vi "runLoopStop.vi"(8 "error in (no error)":errorcluster, 11 "Pixelfly in":refnum<class "Pixelfly.lvclass">) -> (0 "error out":errorcluster, 3 "Pixelfly out":refnum<class "Pixelfly.lvclass">)   [LabVIEW 2011, in "Hardware.lvlib" / "Channels.lvlib" / "Pixelfly.lvclass"]
uses:
  Pixelfly.lvclass
  Pixelfly.lvclass/Pixelfly.ctl
  Tools/Filing/FileSystem/FileSystem.lvclass
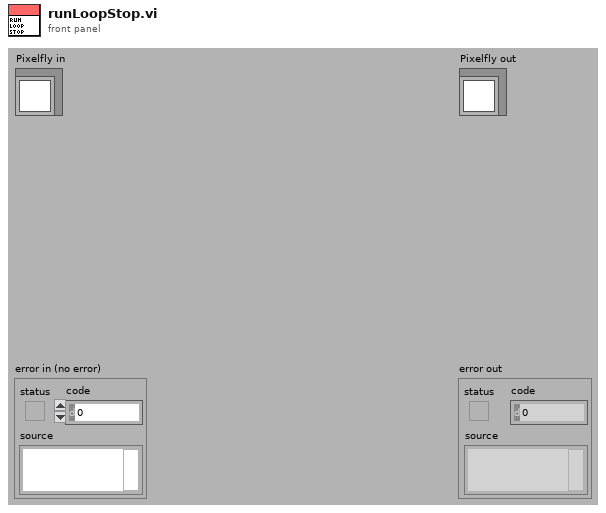
[diagram p1: front panel]
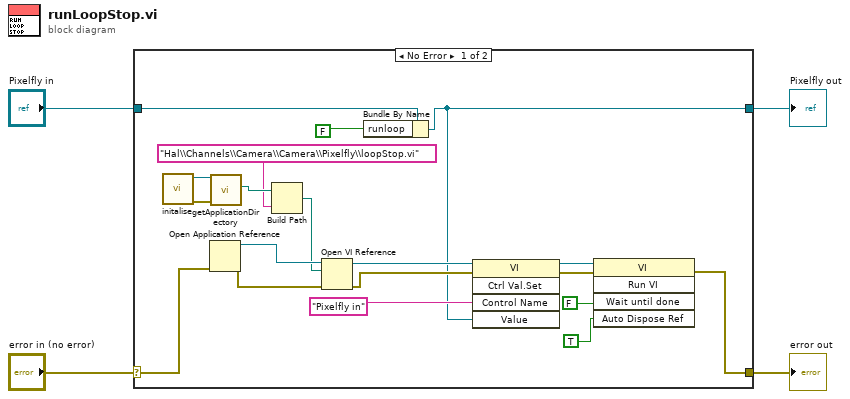
[diagram p0: block diagram]
diagram:
  n1 = case shown="No Error" "error in (no error)" {
    selector: "error in (no error)" -> [w16 w25]
    tunnel: [w8 w25] -> w3
    tunnel: [w6 w24] -> w1
    tunnel: "Pixelfly in" -> [w7 w24]
    frame No Error {
      n2 = call "initalise.vi"() -> ("error out"=w21:errorcluster, "FileSystem out"=w22:refnum<class "FileSystem.lvclass">)  [unwired: 10 in]
      n3 = Open Application Reference(8:w16) -> (0:w17:errorcluster, 3:w23:refnum<vi>)  [unwired: 3 in]
      n4 = call-dynamic "getApplicationDirectory.vi"("error in (no error)"=w21, "FileSystem.lvclass in"=w22) -> ("ApplicationDirectory"=w20:path)  [unwired: 7 in, 2 out]
      n5 = Build Path(base path=w20, name or relative path="Hal\\Channels\\Camera\\Camera\\Pixelfly\\loopStop.vi") -> (appended path=w18:path)
      n6 = Open VI Reference(application reference (local)=w23, vi path=w18, error in (no error)=w17) -> (vi reference=w15:refnum<vi>, error out=w14:errorcluster)  [unwired: 3 in]
      n7 = Bundle By Name(cluster=w7, "runloop"=FALSE) -> (w6:refnum<class "Pixelfly.lvclass">)
      n8 = invoke class="VI" method="Ctrl Val.Set"(reference=w15, error in=w14, "Control Name"="Pixelfly in", "Value"=w6) -> (reference out=w11:refnum<vi>, error out=w12:errorcluster)  [unwired: 1 in, 3 out]
      n9 = invoke class="VI" method="Run VI"(reference=w11, error in=w12, "Wait until done"=FALSE, "Auto Dispose Ref"=TRUE) -> (error out=w8:errorcluster)  [unwired: 1 in, 4 out]
    }
    frame Error {
    }
  }
  "error out" <- w3
  "Pixelfly out" <- w1
